vi "Fit Rabi Pi Pulse.vi"() -> ()   [LabVIEW 2012]
uses:
  <vilib>/Utility/file.llb/Read From Spreadsheet File (DBL).vi
  <vilib>/gmath/NumericalOptimization/Nonlinear Curve Fit LM.vi
  <vilib>/gmath/NI_Gmath.lvlib
panel:
  in  "Rabi data":path=path "C:/Users/Public/Documents/Srujan/2014-06-26/NV2_Rabi_2p8125GHz_m3dBm_switch.txt"
  out "Array":dbl[](array[numeric])=[0.15, 63.0, 0.0, 0.0, 0.0, 0.0, -0.15, -5.0]
  in  "Guess for pi pulse":dbl
  out "Rabi Normalized contrast":cluster{"Y":dbl[], "Y":dbl[]}[](graph)=[{"Y"=[0.012, 0.015310344827586206, 0.018620689655172412, 0.02193103448275862, 0.025241379310344828, 0.02855172413793103, 0.031862068965517236, 0.035172413793103444, 0.03848275862068965, 0.04179310344827586, 0.04510344827586207, 0.048413793103448274, 0.05172413793103448, 0.05503448275862069, 0.0583448275862069, 0.0616551724137931, 0.0649655172413793, 0.0682758620689655, 0.07158620689655172, 0.07489655172413792, 0.07820689655172414, 0.08151724137931034, 0.08482758620689655, 0.08813793103448275, 0.09144827586206897, 0.09475862068965517, 0.09806896551724138, 0.10137931034482758, 0.1046896551724138, 0.108, 0.11131034482758621, 0.11462068965517241, 0.11793103448275863, 0.12124137931034482, 0.12455172413793103, 0.12786206896551724, 0.13117241379310343, 0.13448275862068965, 0.13779310344827586, 0.14110344827586205, 0.14441379310344826, 0.14772413793103448, 0.1510344827586207, 0.15434482758620688, 0.1576551724137931, 0.1609655172413793, 0.16427586206896552, 0.1675862068965517, 0.17089655172413792, 0.17420689655172414, 0.17751724137931035, 0.18082758620689654, 0.18413793103448275, 0.18744827586206897, 0.19075862068965518, 0.19406896551724137, 0.19737931034482759, 0.2006896551724138, 0.204, 0.2073103448275862, 0.21062068965517242, 0.21393103448275863, 0.21724137931034482, 0.22055172413793103, 0.22386206896551725, 0.22717241379310346, 0.23048275862068965, 0.23379310344827586, 0.23710344827586208, 0.24041379310344826, 0.24372413793103445, 0.24703448275862067, 0.25034482758620685, 0.2536551724137931, 0.2569655172413793, 0.2602758620689655, 0.2635862068965517, 0.2668965517241379, 0.27020689655172414, 0.2735172413793103, 0.2768275862068965, 0.28013793103448276, 0.28344827586206894, 0.28675862068965513, 0.2900689655172414, 0.29337931034482756, 0.2966896551724138, 0.3], "Y"=[-0.04069329314242657, -0.09175627240143368, -0.10250737463126836, -0.1041369472182596, -0.1326530612244897, -0.17416131334760881, -0.21134751773049645, -0.28631284916201116, -0.2211336599020295, -0.23330887747615559, -0.24717514124293793, -0.15837796480489677, -0.2288888888888888, -0.19809244314013202, -0.22746781115879822, -0.2178289000718907, -0.24873463485177152, -0.19629629629629627, -0.22723908216136196, -0.18337218337218333, -0.22245762711864406, -0.21386861313868616, -0.19219440353460968, -0.15828402366863914, -0.17686072218128232, -0.1615720524017467, -0.1755780346820809, -0.16607773851590105, -0.17273376159885798, -0.17988668555240797, -0.08751902587519025, -0.144561403508772, -0.10611643330876937, -0.05519244734930999, -0.0967741935483871, -0.08202567760342368, -0.05878030859662016, -0.11530398322851156, -0.02666666666666661, -0.05982905982905986, -0.0817790530846484, -0.06971830985915502, -0.024630541871921156, 0.014136904761904701, 0.0014609203798392392, 0.03252032520325199, -0.012587412587412559, 0.030124908155767738, 0.013148283418553659, 0.0806451612903226, 0.013768115942029053, 0.06661786237188867, 0.05203619909502273, -0.03856749311294764, -0.0029651593773165385, 0.019636363636363594, 0.00670141474311255, -0.021276595744680875, 0.004360465116279144, 0.024924471299093687, -0.08573436401967666, -0.05029154518950435, -0.02552881108679793, -0.0648148148148149, -0.10436713545521835, -0.09770114942528736, -0.05377147124719941, -0.13543859649122814, -0.11997019374068557, -0.16049382716049373, -0.10194902548725639, -0.13120830244625653, -0.161504424778761, -0.1736311239193084, -0.18084345961401008, -0.21134020618556695, -0.22222222222222218, -0.2334047109207709, -0.2154065620542083, -0.25215517241379304, -0.15744680851063828, -0.2404795486600846, -0.24043321299638987, -0.1862955032119914, -0.20865862313697658, -0.22429906542056083, -0.19926739926739928, -0.2138769670958512]}]
  in  "Enum":T1(ring)
  # "UNFINISHED"
  # "ns"
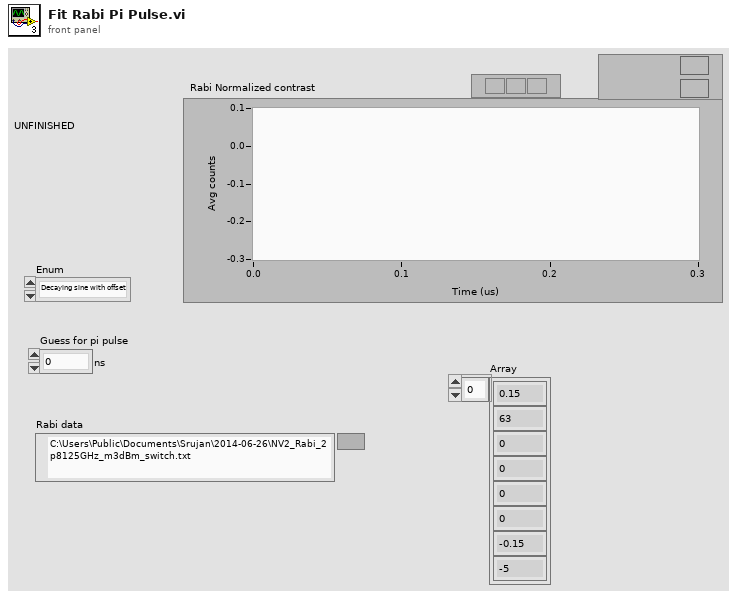
[diagram p1: front panel]
types:
  T1 = enum16{"Decaying sine with offset", "Sine with offset", "Sum of 2 sines"}
  T2 = cluster{"all rows":dbl[], "best nonlinear fit":dbl[]}
  T3 = cluster{"all rows":dbl[], "best nonlinear fit":dbl[]}[]
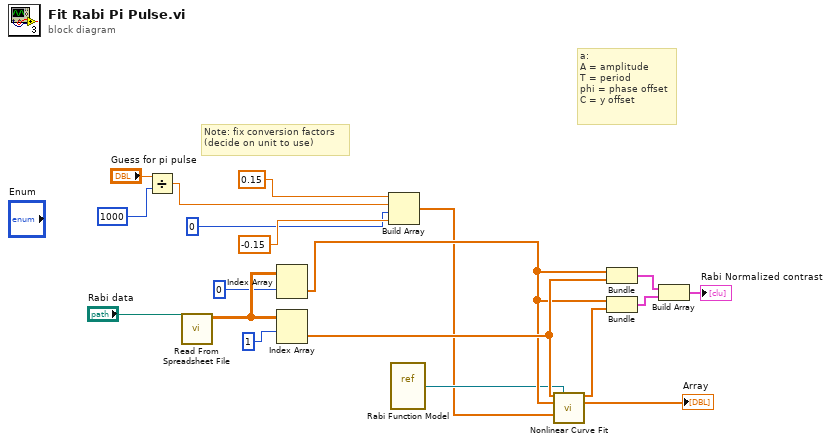
[diagram p0: block diagram]
diagram:
  # "a:\nA = amplitude\nT = period\nphi = phase offset\nC = y offset"
  # "Note: fix conversion factors\n(decide on unit to use)"
  n1 = Divide(x="Guess for pi pulse", y=1000) -> (x/y=w1:dbl)
  n2 = call-poly <vilib>:"Read From Spreadsheet File.vi"("file path (dialog if empty)"="Rabi data") -> ("all rows"=w13:dbl[][])  [unwired: 6 in, 4 out]
  n3 = Index Array(array=w13, index (row)=0) -> (element=w10:dbl[])  [unwired: 1 in]
  n4 = Index Array(array=w13, index (row)=1) -> (element=w11:dbl[])  [unwired: 1 in]
  n5 = Build Array(0.15, w1, 0, -0.15) -> (w4:dbl[])
  n6 = vi-ref "Rabi Function Model.vi"() -> (w8:refnum<vi>)
  n7 = call-poly <vilib>:"Nonlinear Curve Fit.vi"("Y"=w11, "f(x,a)"=w8, "X"=w10, "initial parameters"=w4) -> ("best nonlinear fit"=w9:dbl[], "best fit parameters"=→"Array":dbl[])  [unwired: 6 in, 4 out]
  n8 = Bundle("all rows"=w10, "all rows"=w11) -> (w16:cluster{"all rows":dbl[], "all rows":dbl[]})  [unwired: 1 in]
  n9 = Bundle("all rows"=w10, "best nonlinear fit"=w9) -> (w18:T2)  [unwired: 1 in]
  n10 = Build Array(w16, w18) -> (→"Rabi Normalized contrast":T3)
